vi "DEAB Open LV80 Project App Reference.vi"(1 "close ref? (false)":bool) -> (0 "App Ref":refnum<vi>)   [LabVIEW 2011]
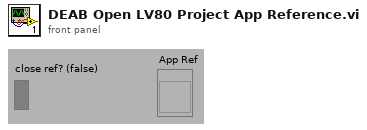
[diagram p1: front panel]
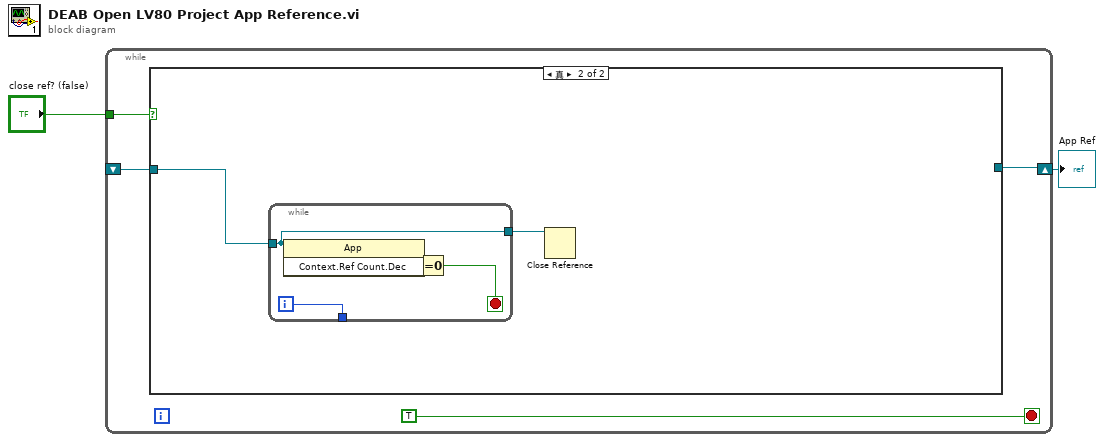
[diagram p0: block diagram]
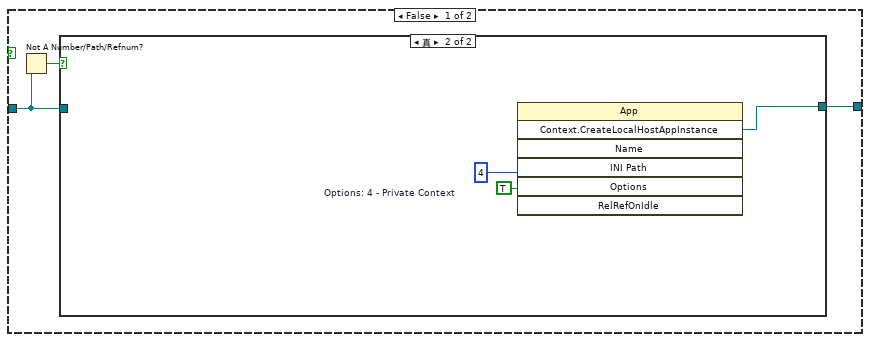
[diagram p2: hidden frame]
diagram:
  n1 = while {
    shift-right: [w6] -> w2
    shift-left: _ -> [w5]
    tunnel: "close ref? (false)" -> [w3]
    stop <- TRUE stop-if-true
    n2 = case shown="真" w3 {
      tunnel: [w9 _] -> w6
      tunnel: w5 -> [w7 w14]
      frame False {
        n3 = Not A Number/Path/Refnum?(number/path/refnum=w7) -> (NaN/Path/Refnum?=w8:bool)
        n4 = case shown="真" w8 {
          tunnel: [w10 w13] -> w9
          tunnel: w7 -> [w10 _]
          frame False {
          }
          frame True {
            w12 = 4  # Options: 4 - Private Context
            n5 = invoke class="App" method="Context.CreateLocalHostAppInstance"("Options"=w12, "RelRefOnIdle"=TRUE ("Release Ref on Idle (T)")) -> ("Create Context"=w13:refnum<vi>)  [unwired: 5 in, 6 out]
          }
        }
      }
      frame True {
        n6 = while {
          tunnel: w14 -> [w17]
          tunnel: [w17] -> w15
          tunnel: [w16] -> _
          i -> [w16]
          stop <- w18 stop-if-true
          n7 = invoke class="App" method="Context.Ref Count.Dec"(reference=w17) -> ("Context.Ref Count.Dec"=w19:i32)  [unwired: 2 in, 2 out]
          n8 = Equal To 0?(x=w19) -> (x = 0?=w18:bool)
        }
        n9 = Close Reference(reference=w15) -> ()  [unwired: 1 in, 1 out]
      }
    }
  }
  "App Ref" <- w2
